vi "Day03-02_자판기.vi"() -> ()   [LabVIEW 2021]
panel:
  out "배출 상품명(문자형)":string
  out "현재 잔액(숫자형)":dbl
  in  "정지 버튼":bool
  in  "거스름돈 반환":bool
  in  "1000원":bool
  in  "500원":bool
  out "웰치스 LED":bool
  in  "웰치스":bool
  in  "100원":bool
  out "콜라 LED":bool
  in  "콜라":bool
  in  "50원":bool
  out "환타 LED":bool
  in  "환타":bool
  in  "10원":bool
  out "사이다 LED":bool
  in  "사이다":bool
  # "900원"
  # "1000원"
  # "1100원"
  # "1200원"
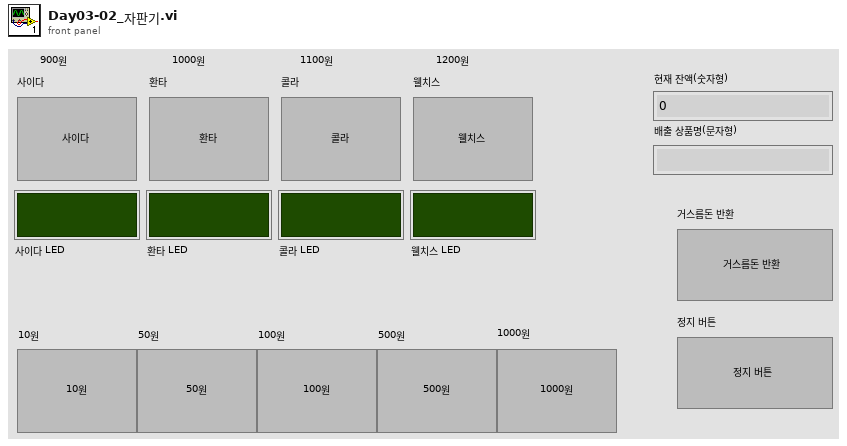
[diagram p1: front panel]
types:
  T1 = typedef "자판기 상태 열거형 상수.ctl" = enum16{"초기화", "대기", "콜라", "사이다", "환타", "웰치스", "10원", "50원", "100원", "500원", "1000원", "LED 업데이트", "잔돈반환", "정지"}
  T2 = cluster{"상태":T1, "사이다 LED":bool, "환타 LED":bool, "콜라 LED":bool, "웰치스 LED":bool, "현재 잔액":dbl, "배출 상품명":string}
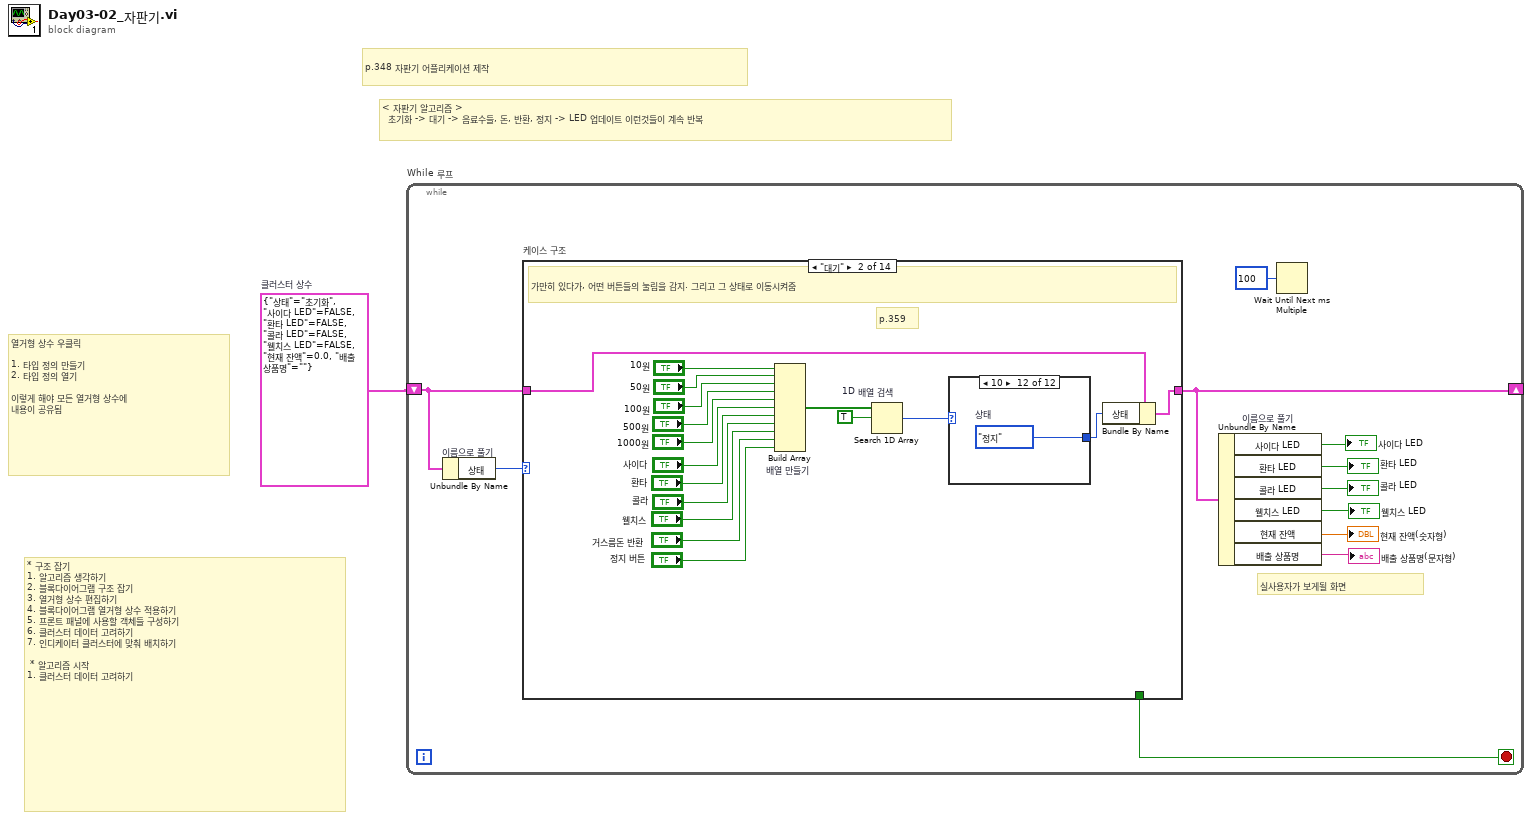
[diagram p0: block diagram]
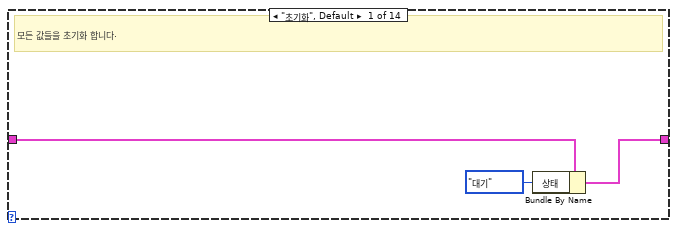
[diagram p2: hidden frame]
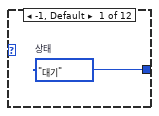
[diagram p3: hidden frame]
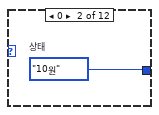
[diagram p4: hidden frame]
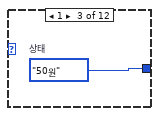
[diagram p5: hidden frame]
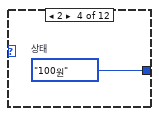
[diagram p6: hidden frame]
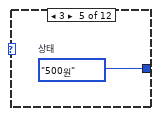
[diagram p7: hidden frame]
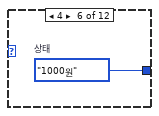
[diagram p8: hidden frame]
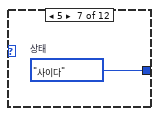
[diagram p9: hidden frame]
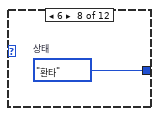
[diagram p10: hidden frame]
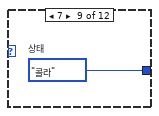
[diagram p11: hidden frame]
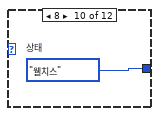
[diagram p12: hidden frame]
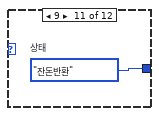
[diagram p13: hidden frame]
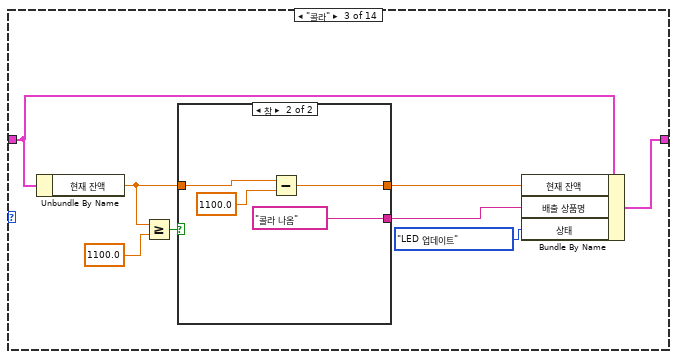
[diagram p14: hidden frame]
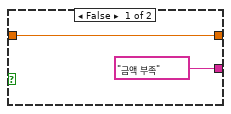
[diagram p15: hidden frame]
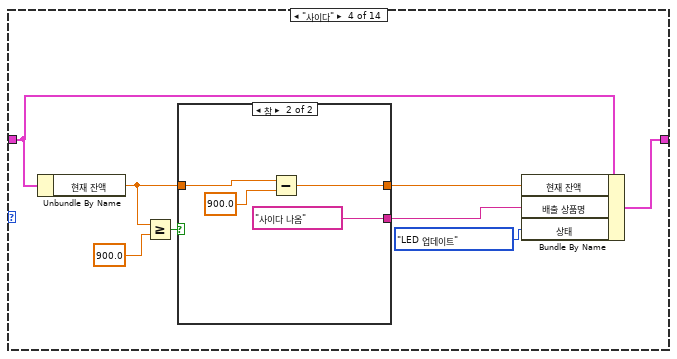
[diagram p16: hidden frame]
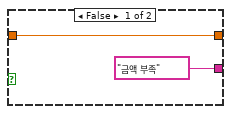
[diagram p17: hidden frame]
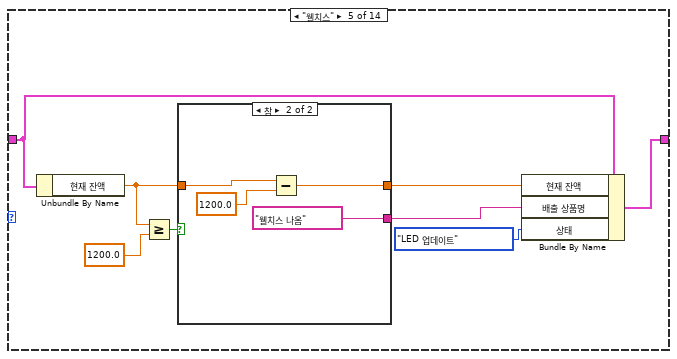
[diagram p18: hidden frame]
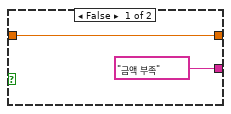
[diagram p19: hidden frame]
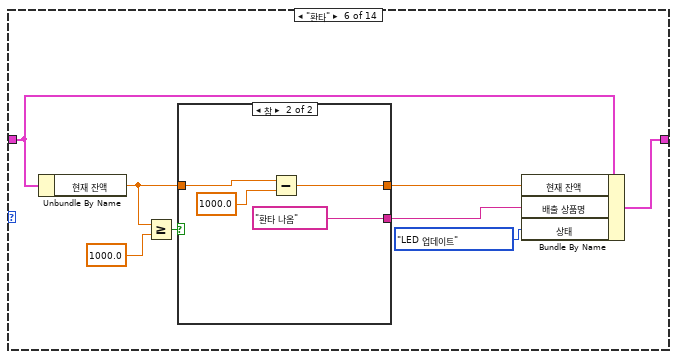
[diagram p20: hidden frame]
diagram:
  w1 = T2 {"상태"=enum."초기화", "사이다 LED"=FALSE, "환타 LED"=FALSE, "콜라 LED"=FALSE, "웰치스 LED"=FALSE, "현재 잔액"=0.0, "배출 상품명"=""}  # 클러스터 상수
  # "* 구조 잡기\n1. 알고리즘 생각하기\n2. 블록다이어그램 구조 잡기\n3. 열거형 상수 편집하기\n4. 블록다이어그램 열거형 상수 적용하기\n5. 프론트 패널에 사용할 객체들 구성하기\n6. 클러스터 데이터 고려하기\n7. 인디케이터 클러스터에 맞춰 배치하기\n\n * 알고리즘 시작\n1. 클러스터 데이터 고려하기"
  # "열거형 상수 우클릭\n\n1. 타입 정의 만들기\n2. 타입 정의 열기\n\n이렇게 해야 모든 열거형 상수에\n내용이 공유됨"
  # "< 자판기 알고리즘 >\n  초기화 -> 대기 -> 음료수들, 돈, 반환, 정지 -> LED 업데이트 이런것들이 계속 반복"
  # "p.348 자판기 어플리케이션 제작"
  n1 = while "While 루프" {
    shift-right: [w10] -> _
    shift-left: w1 -> [w11]
    stop <- w3 stop-if-true
    # "실사용자가 보게될 화면"
    n2 = Unbundle By Name "이름으로 풀기"(w11) -> ("상태"=w12:T1)
    n3 = case "케이스 구조" shown="\"대기\"" w12 {
      tunnel: w11 -> [w15 w18 w51 w65 w79 w93 w102 w108 w114 w120 w127 w141 w148 _]
      tunnel: [w14 w16 w50 w64 w78 w92 w101 w107 w113 w119 w126 w140 w144 _] -> w10
      tunnel: [_ _ _ _ _ _ _ _ _ _ _ _ _ TRUE] -> w3
      frame "초기화", Default {
        # "모든 값들을 초기화 합니다."
        n4 = Bundle By Name(cluster=w15, "상태"=자판기_상태_열거형_상수."대기") -> (w14:T2)
      }
      frame "대기" {
        # "p.359"
        # "가만히 있다가, 어떤 버튼들의 눌림을 감지. 그리고 그 상태로 이동시켜줌"
        n5 = Build Array "배열 만들기"("10원", "50원", "100원", "500원", "1000원", "사이다", "환타", "콜라", "웰치스", "거스름돈 반환", "정지 버튼") -> (w21:bool[])
        n6 = Search 1D Array "1D 배열 검색"(1D array=w21, element=TRUE) -> (index of element=w19:i32)  [unwired: 1 in]
        n7 = case shown="10" w19 {
          tunnel: [w33 w34 w35 w36 w37 w38 w39 w40 w41 w42 w43 w44] -> w17
          frame -1, Default {
            w33 = 자판기_상태_열거형_상수."대기"  # 상태
          }
          frame 0 {
            w34 = 자판기_상태_열거형_상수."10원"  # 상태
          }
          frame 1 {
            w35 = 자판기_상태_열거형_상수."50원"  # 상태
          }
          frame 2 {
            w36 = 자판기_상태_열거형_상수."100원"  # 상태
          }
          frame 3 {
            w37 = 자판기_상태_열거형_상수."500원"  # 상태
          }
          frame 4 {
            w38 = 자판기_상태_열거형_상수."1000원"  # 상태
          }
          frame 5 {
            w39 = 자판기_상태_열거형_상수."사이다"  # 상태
          }
          frame 6 {
            w40 = 자판기_상태_열거형_상수."환타"  # 상태
          }
          frame 7 {
            w41 = 자판기_상태_열거형_상수."콜라"  # 상태
          }
          frame 8 {
            w42 = 자판기_상태_열거형_상수."웰치스"  # 상태
          }
          frame 9 {
            w43 = 자판기_상태_열거형_상수."잔돈반환"  # 상태
          }
          frame 10 {
            w44 = 자판기_상태_열거형_상수."정지"  # 상태
          }
        }
        n8 = Bundle By Name(cluster=w18, "상태"=w17) -> (w16:T2)
      }
      frame "콜라" {
        n9 = Unbundle By Name(w51) -> ("현재 잔액"=w48:dbl)
        n10 = Greater Or Equal?(x=w48, y=1100.0) -> (x >= y?=w49:bool)
        n11 = case shown="참" w49 {
          tunnel: w48 -> [w54 w58]
          tunnel: [w54 w56] -> w47
          tunnel: ["금액 부족" "콜라 나옴"] -> w46
          frame False {
          }
          frame True {
            n12 = Subtract(x=w58, y=1100.0) -> (x-y=w56:dbl)
          }
        }
        n13 = Bundle By Name(cluster=w51, "현재 잔액"=w47, "배출 상품명"=w46, "상태"=자판기_상태_열거형_상수."LED 업데이트") -> (w50:T2)
      }
      frame "사이다" {
        n14 = Unbundle By Name(w65) -> ("현재 잔액"=w62:dbl)
        n15 = Greater Or Equal?(x=w62, y=900.0) -> (x >= y?=w63:bool)
        n16 = case shown="참" w63 {
          tunnel: w62 -> [w68 w72]
          tunnel: [w68 w70] -> w61
          tunnel: ["금액 부족" "사이다 나옴"] -> w60
          frame False {
          }
          frame True {
            n17 = Subtract(x=w72, y=900.0) -> (x-y=w70:dbl)
          }
        }
        n18 = Bundle By Name(cluster=w65, "현재 잔액"=w61, "배출 상품명"=w60, "상태"=자판기_상태_열거형_상수."LED 업데이트") -> (w64:T2)
      }
      frame "웰치스" {
        n19 = Unbundle By Name(w79) -> ("현재 잔액"=w76:dbl)
        n20 = Greater Or Equal?(x=w76, y=1200.0) -> (x >= y?=w77:bool)
        n21 = case shown="참" w77 {
          tunnel: w76 -> [w82 w86]
          tunnel: [w82 w84] -> w75
          tunnel: ["금액 부족" "웰치스 나옴"] -> w74
          frame False {
          }
          frame True {
            n22 = Subtract(x=w86, y=1200.0) -> (x-y=w84:dbl)
          }
        }
        n23 = Bundle By Name(cluster=w79, "현재 잔액"=w75, "배출 상품명"=w74, "상태"=자판기_상태_열거형_상수."LED 업데이트") -> (w78:T2)
      }
      frame "환타" {
        n24 = Unbundle By Name(w93) -> ("현재 잔액"=w90:dbl)
        n25 = Greater Or Equal?(x=w90, y=1000.0) -> (x >= y?=w91:bool)
        n26 = case shown="참" w91 {
          tunnel: w90 -> [w96 w100]
          tunnel: [w96 w98] -> w89
          tunnel: ["금액 부족" "환타 나옴"] -> w88
          frame False {
          }
          frame True {
            n27 = Subtract(x=w100, y=1000.0) -> (x-y=w98:dbl)
          }
        }
        n28 = Bundle By Name(cluster=w93, "현재 잔액"=w89, "배출 상품명"=w88, "상태"=자판기_상태_열거형_상수."LED 업데이트") -> (w92:T2)
      }
      frame "10원" {
        # "현재잔액에서 10원을 더해줍니다."
        n29 = Unbundle By Name(w102) -> ("현재 잔액"=w105:dbl)
        n30 = Add(x=w105, y=10.0) -> (x+y=w106:dbl)
        n31 = Bundle By Name(cluster=w102, "현재 잔액"=w106, "상태"=자판기_상태_열거형_상수."LED 업데이트") -> (w101:T2)
      }
      frame "50원" {
        # "현재잔액에서 50원원을 더해줍니다."
        n32 = Unbundle By Name(w108) -> ("현재 잔액"=w112:dbl)
        n33 = Add(x=w112, y=50.0) -> (x+y=w111:dbl)
        n34 = Bundle By Name(cluster=w108, "현재 잔액"=w111, "상태"=자판기_상태_열거형_상수."LED 업데이트") -> (w107:T2)
      }
      frame "100원" {
        # "현재잔액에서 100원원을 더해줍니다."
        n35 = Unbundle By Name(w114) -> ("현재 잔액"=w117:dbl)
        n36 = Add(x=w117, y=100.0) -> (x+y=w118:dbl)
        n37 = Bundle By Name(cluster=w114, "현재 잔액"=w118, "상태"=자판기_상태_열거형_상수."LED 업데이트") -> (w113:T2)
      }
      frame "500원" {
        # "현재잔액에서 500원을 더해줍니다."
        n38 = Unbundle By Name(w120) -> ("현재 잔액"=w124:dbl)
        n39 = Add(x=w124, y=500.0) -> (x+y=w123:dbl)
        n40 = Bundle By Name(cluster=w120, "현재 잔액"=w123, "상태"=자판기_상태_열거형_상수."LED 업데이트") -> (w119:T2)
      }
      frame "1000원" {
        # "현재잔액에서 1000원원을 더해줍니다."
        n41 = Unbundle By Name(w127) -> ("현재 잔액"=w130:dbl)
        n42 = Add(x=w130, y=1000.0) -> (x+y=w128:dbl)
        n43 = Bundle By Name(cluster=w127, "현재 잔액"=w128, "상태"=자판기_상태_열거형_상수."LED 업데이트") -> (w126:T2)
      }
      frame "LED 업데이트" {
        n44 = Unbundle By Name(w141) -> ("현재 잔액"=w134:dbl)
        n45 = Greater Or Equal?(x=w134, y=900.0) -> (x >= y?=w139:bool)
        n46 = Greater Or Equal?(x=w134, y=1000.0) -> (x >= y?=w133:bool)
        n47 = Greater Or Equal?(x=w134, y=1100.0) -> (x >= y?=w132:bool)
        n48 = Greater Or Equal?(x=w134, y=1200.0) -> (x >= y?=w131:bool)
        n49 = Bundle By Name(cluster=w141, "사이다 LED"=w139, "환타 LED"=w133, "콜라 LED"=w132, "웰치스 LED"=w131, "상태"=자판기_상태_열거형_상수."대기") -> (w140:T2)
      }
      frame "잔돈반환" {
        n50 = Bundle By Name(cluster=w148, "상태"=자판기_상태_열거형_상수."대기", "현재 잔액"=0.0, "배출 상품명"="잔돈이 반환되었습니다.", "상태"=자판기_상태_열거형_상수."LED 업데이트") -> (w144:T2)
      }
      frame "정지" {
      }
    }
    n51 = Unbundle By Name "이름으로 풀기"(w10) -> ("사이다 LED"=→"사이다 LED":bool, "환타 LED"=→"환타 LED":bool, "콜라 LED"=→"콜라 LED":bool, "웰치스 LED"=→"웰치스 LED":bool, "현재 잔액"=→"현재 잔액(숫자형)":dbl, "배출 상품명"=→"배출 상품명(문자형)":string)
    n52 = Wait Until Next ms Multiple(millisecond multiple=u32 100 ("ms 배수")) -> ()  [unwired: 1 out]
  }
